vi "Terminal-Core-ModbusModule.vi"(0 "ModbusNReqRef":refnum<notifier>, 5 "ModbusNResRef":refnum<notifier>, 7 "ModbusMsgQRef":refnum<queue>, 9 "GuiModbusQRef":refnum<queue>, 11 "error in":errorcluster, 12 "ErrorQRef":refnum<queue>) -> (15 "error out":errorcluster)   [LabVIEW 2014]
panel:
  out "Exception Code":u8 format="%.0x"
  out "Holding Registers":u16[](array[numeric])
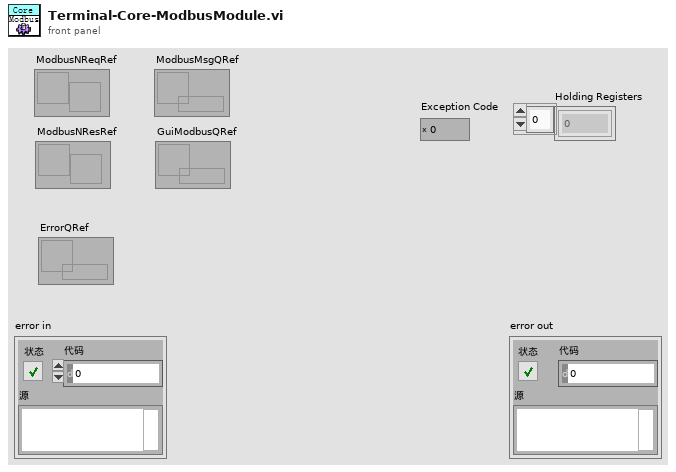
[diagram p1: front panel]
types:
  T1 = cluster{"Transaction ID":u16, "Unit ID":u8, "Starting Address":u16, "Quantity":u16}
  T2 = cluster{"Transaction ID":u16, "Unit ID":u8, "Address":u16, "Register":u16}
  T3 = cluster{"Transaction ID":u16, "Unit ID":u8, "Starting Address":u16, "Registers":u16[]}
  T4 = cluster{"Transaction ID":u16, "Unit ID":u8, "Starting Address":u16, "Quantity":u16, "Holding Registers":u16[], "Exception Code":u8}
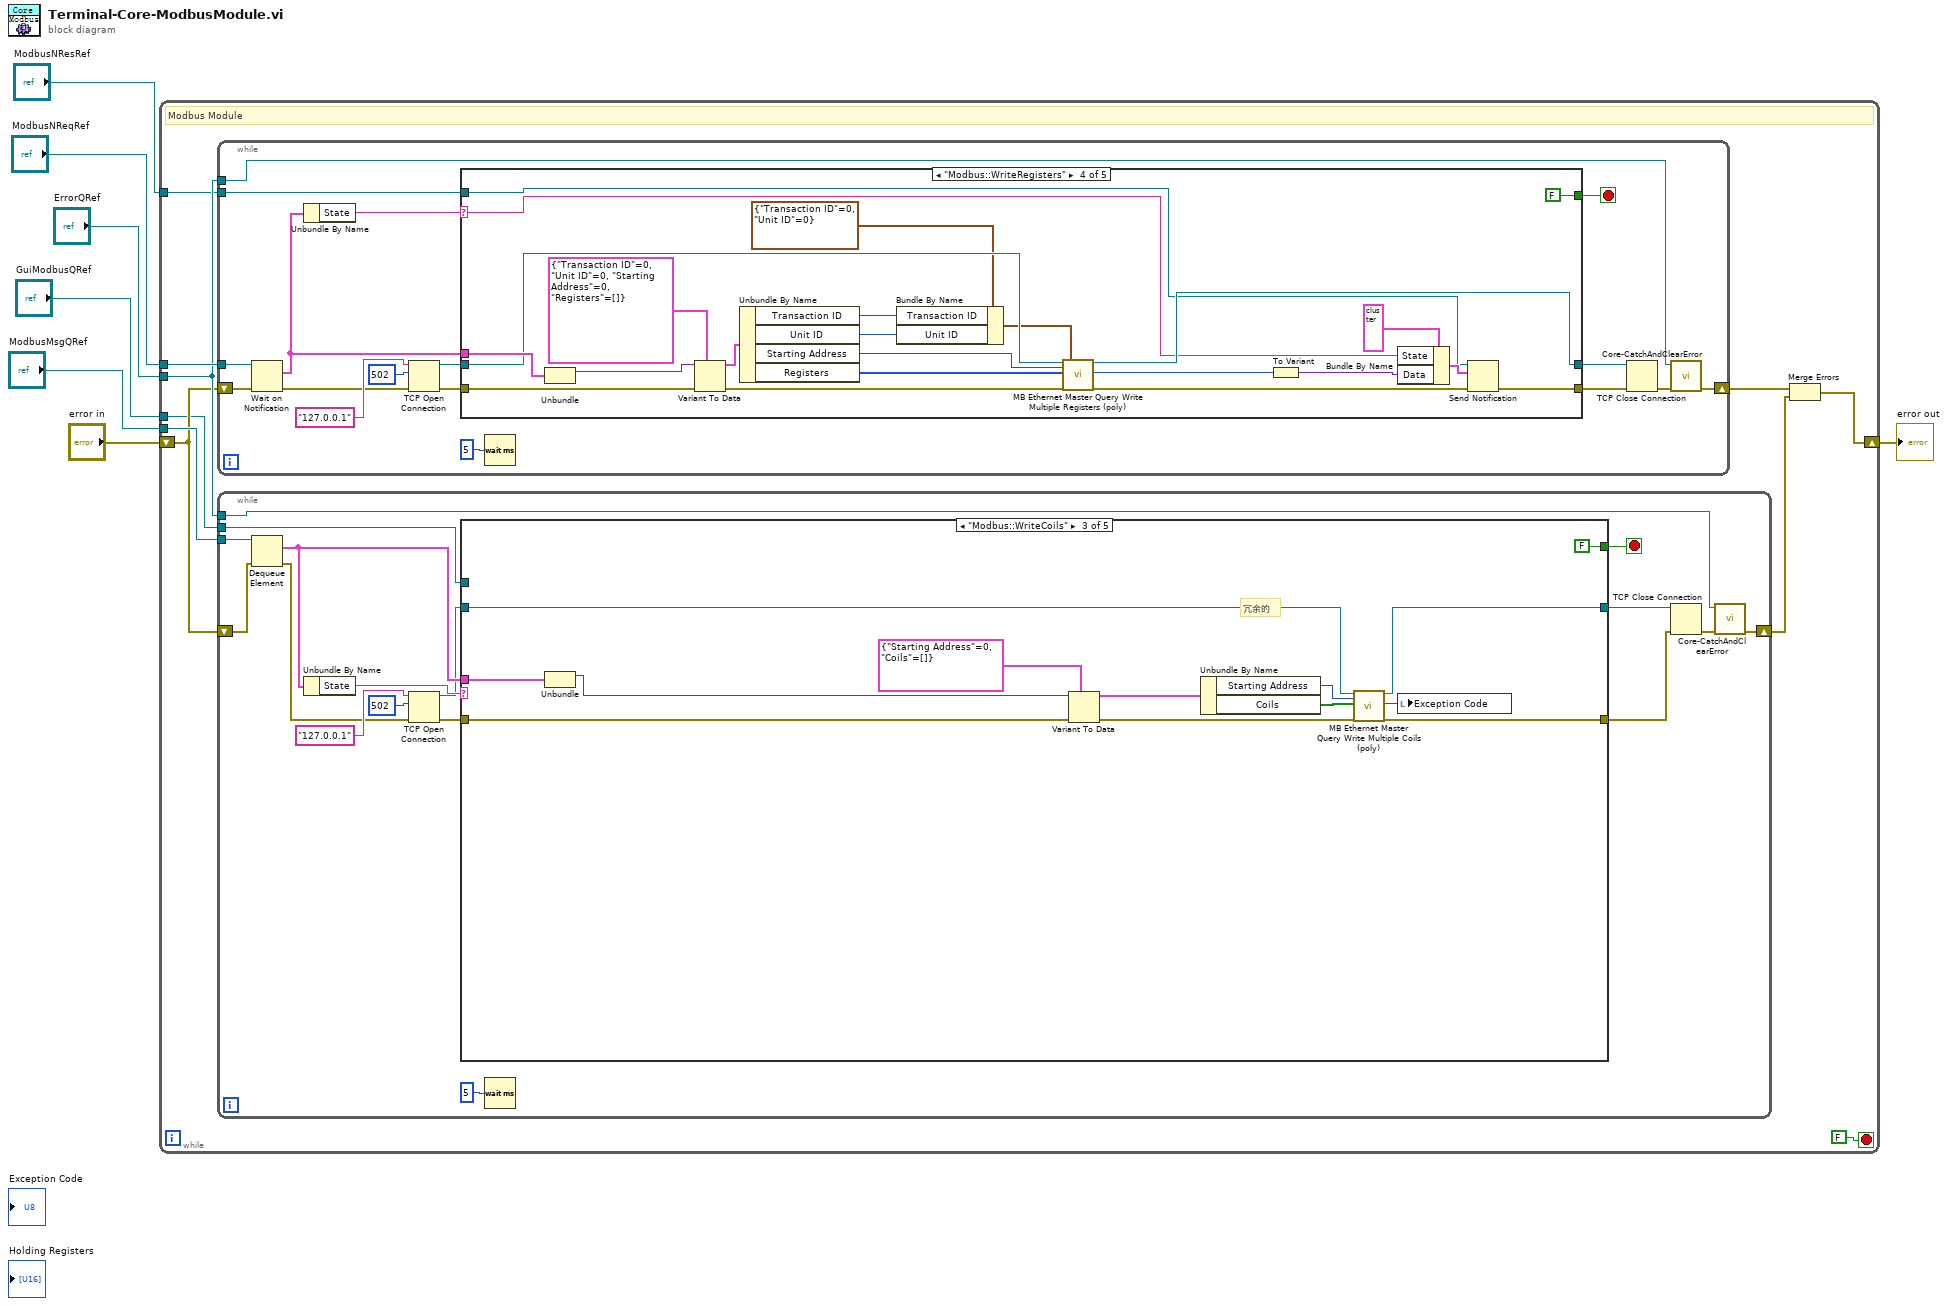
[diagram p0: block diagram]
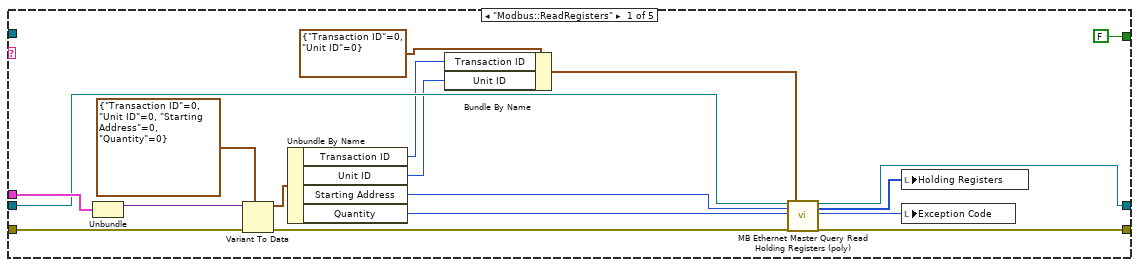
[diagram p2: hidden frame]
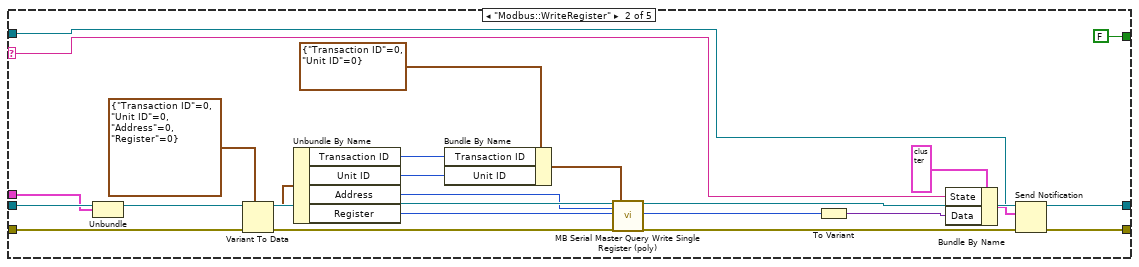
[diagram p3: hidden frame]
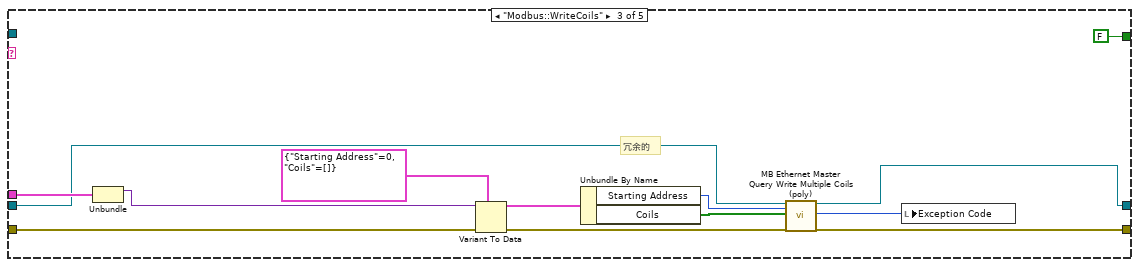
[diagram p4: hidden frame]
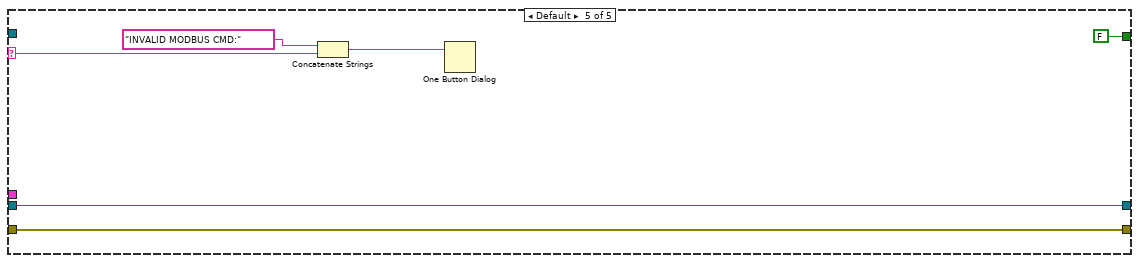
[diagram p5: hidden frame]
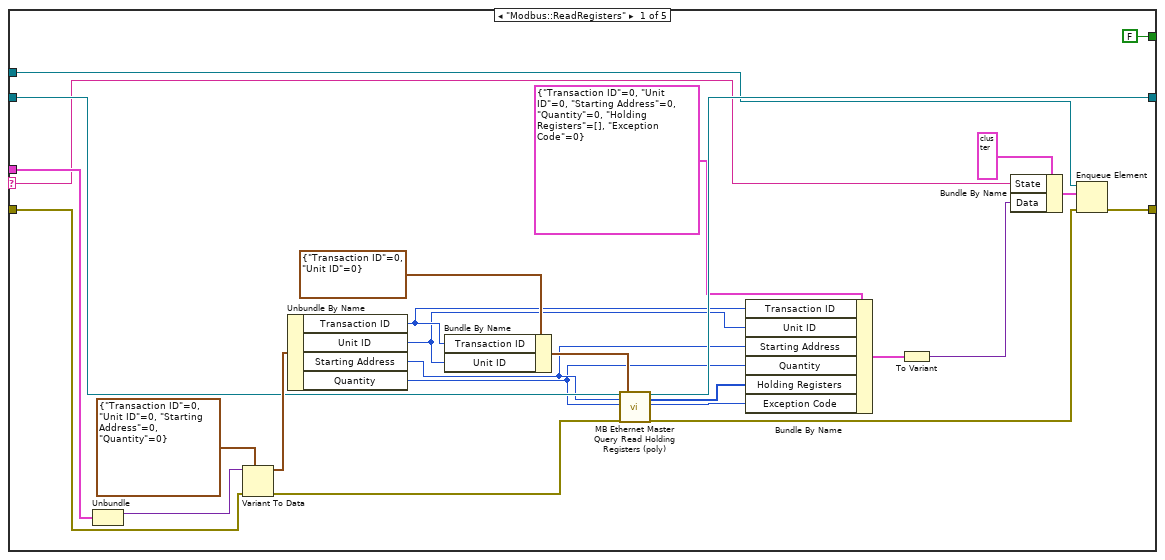
[diagram p6: hidden frame]
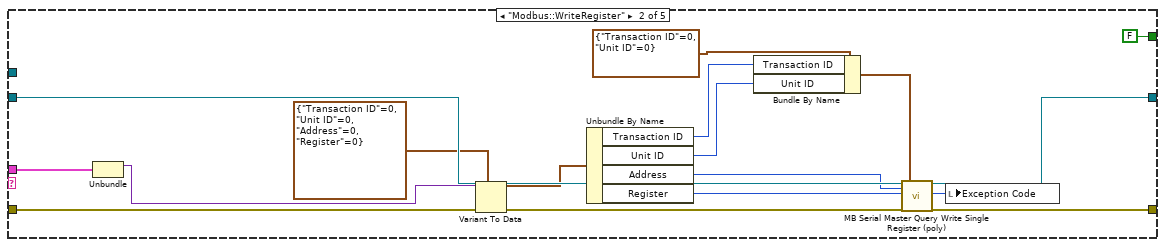
[diagram p7: hidden frame]
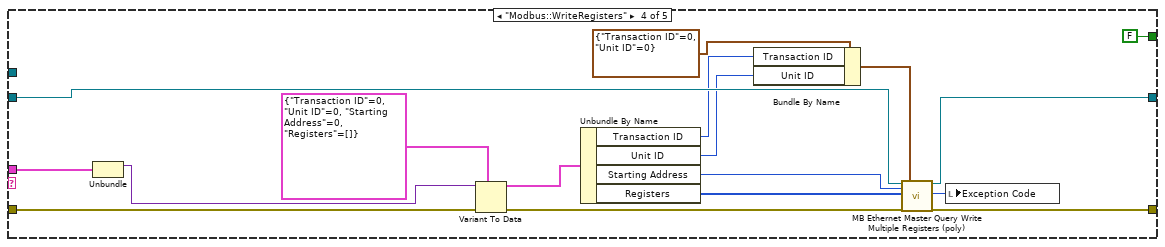
[diagram p8: hidden frame]
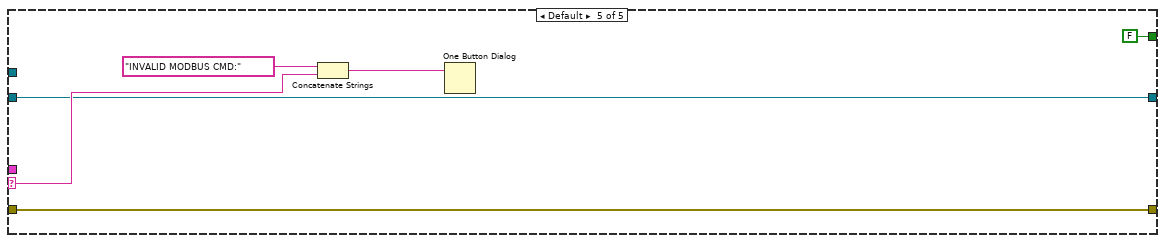
[diagram p9: hidden frame]
diagram:
  n1 = while {
    shift-right: [w8] -> w4
    shift-left: "error in" -> [w13]
    tunnel: "ErrorQRef" -> [w14]
    tunnel: "ModbusMsgQRef" -> [w17]
    tunnel: "ModbusNReqRef" -> [w15]
    tunnel: "ModbusNResRef" -> [w12]
    tunnel: "GuiModbusQRef" -> [w11]
    stop <- FALSE stop-if-true
    # "Modbus Module"
    n2 = while {
      tunnel: w14 -> [w34]
      shift-right: [w33] -> w10
      shift-left: w13 -> [w21]
      tunnel: w15 -> [w20]
      tunnel: w12 -> [w18]
      stop <- w24 stop-if-true
      n3 = Wait on Notification(notifier=w20, error in (no error)=w21) -> (notification=w19:cluster{"Data":variant, "State":string}, error out=w22:errorcluster)  [unwired: 2 in, 2 out]
      n4 = Unbundle By Name(w19) -> ("State"=w32:string)
      n5 = TCP Open Connection(address="127.0.0.1" ("地址"), remote port or service name=u16 502 ("远程端口或服务名称"), error in (no error)=w22) -> (connection ID=w28:refnum<k5>, error out=w29:errorcluster)  [unwired: 2 in]
      n6 = case shown="\"Modbus::WriteRegisters\"" w32 {
        selector: w32 -> [_ w58 _ w94 w115]
        tunnel: w19 -> [w52 w72 w87 w107 _]
        tunnel: w18 -> [_ w60 _ w91 _]
        tunnel: [FALSE FALSE FALSE FALSE FALSE] -> w24
        tunnel: w29 -> [w43 w73 w84 w106 w112]
        tunnel: w28 -> [w46 w74 w85 w104 w113]
        tunnel: [w45 w67 w81 w103 w113] -> w27
        tunnel: [w44 w54 w82 w89 w112] -> w26
        frame "Modbus::ReadRegisters" {
          n7 = Unbundle(w52) -> ("Data"=w51:variant)  [unwired: 1 out]
          n8 = Variant To Data(error in=w43, type=T1 {"Transaction ID"=0, "Unit ID"=0, "Starting Address"=0, "Quantity"=0}, Variant=w51) -> (data=w49:T1, error out=w42:errorcluster)
          n9 = Unbundle By Name(w49) -> ("Transaction ID"=w36:u16, "Unit ID"=w35:u8, "Starting Address"=w38:u16, "Quantity"=w37:u16)
          n10 = Bundle By Name(cluster=cluster{"Transaction ID":u16, "Unit ID":u8} {"Transaction ID"=0, "Unit ID"=0} ("MBAP Header"), "Transaction ID"=w36, "Unit ID"=w35) -> (w39:cluster{"Transaction ID":u16, "Unit ID":u8})
          n11 = call "MB Ethernet Master Query Read Holding Registers (poly).vi"("TCP Connection Refnum in"=w46, "Starting Address"=w38, "Quantity"=w37, "error in"=w42, "MBAP Header"=w39) -> ("TCP Connection Refnum (dup)"=w45:refnum<k5>, "Holding Registers"=w47:u16[], "Exception Code"=w48:u8, "error out"=w44:errorcluster)  [unwired: 11 in]
          n12 = local write "Holding Registers"(w47) -> ()
          n13 = local write "Exception Code"(w48) -> ()
        }
        frame "Modbus::WriteRegister" {
          n14 = Unbundle(w72) -> ("Data"=w71:variant)  [unwired: 1 out]
          n15 = Variant To Data(error in=w73, type=T2 {"Transaction ID"=0, "Unit ID"=0, "Address"=0, "Register"=0}, Variant=w71) -> (data=w69:T2, error out=w68:errorcluster)
          n16 = Unbundle By Name(w69) -> ("Transaction ID"=w64:u16, "Unit ID"=w63:u8, "Address"=w62:u16, "Register"=w61:u16)
          n17 = Bundle By Name(cluster=cluster{"Transaction ID":u16, "Unit ID":u8} {"Transaction ID"=0, "Unit ID"=0} ("MBAP Header"), "Transaction ID"=w64, "Unit ID"=w63) -> (w65:cluster{"Transaction ID":u16, "Unit ID":u8})
          n18 = call "MB Serial Master Query Write Single Register (poly).vi"("VISA resource name"=w74, "Address"=w62, "Holding Register"=w61, "error in"=w68, "Serial Parameters"=w65) -> ("VISA resource name out"=w67:refnum<visa-resource-name>, "Exception Code"=w57:u8, "error out"=w55:errorcluster)  [unwired: 12 in]
          n19 = To Variant(anything=w57) -> (Variant=w56:variant)
          n20 = Bundle By Name(cluster=cluster{"Data":variant, "State":string} {"Data"=variant, "State"=""} ("通知"), "State"=w58, "Data"=w56) -> (w53:cluster{"Data":variant, "State":string})
          n21 = Send Notification(notification=w53, notifier=w60, error in (no error)=w55) -> (error out=w54:errorcluster)  [unwired: 1 out]
        }
        frame "Modbus::WriteCoils" {
          # "冗余的"
          n22 = Unbundle(w87) -> ("Data"=w86:variant)  [unwired: 1 out]
          n23 = Variant To Data(error in=w84, type=cluster{"Starting Address":u16, "Coils":bool[]} {"Starting Address"=0, "Coils"=[]}, Variant=w86) -> (data=w78:cluster{"Starting Address":u16, "Coils":bool[]}, error out=w83:errorcluster)
          n24 = Unbundle By Name(w78) -> ("Starting Address"=w77:u16, "Coils"=w76:bool[])
          n25 = call "MB Ethernet Master Query Write Multiple Coils (poly).vi"("TCP Connection Refnum in"=w85, "Starting Address"=w77, "Coils"=w76, "error in"=w83) -> ("TCP Connection Refnum (dup)"=w81:refnum<k5>, "Exception Code"=w80:u8, "error out"=w82:errorcluster)  [unwired: 13 in]
          n26 = local write "Exception Code"(w80) -> ()
        }
        frame "Modbus::WriteRegisters" {
          n27 = Unbundle(w107) -> ("Data"=w110:variant)  [unwired: 1 out]
          n28 = Variant To Data(error in=w106, type=T3 {"Transaction ID"=0, "Unit ID"=0, "Starting Address"=0, "Registers"=[]}, Variant=w110) -> (data=w108:T3, error out=w105:errorcluster)
          n29 = Unbundle By Name(w108) -> ("Transaction ID"=w99:u16, "Unit ID"=w98:u8, "Starting Address"=w101:u16, "Registers"=w102:u16[])
          n30 = Bundle By Name(cluster=cluster{"Transaction ID":u16, "Unit ID":u8} {"Transaction ID"=0, "Unit ID"=0} ("MBAP Header"), "Transaction ID"=w99, "Unit ID"=w98) -> (w97:cluster{"Transaction ID":u16, "Unit ID":u8})
          n31 = call "MB Ethernet Master Query Write Multiple Registers (poly).vi"("TCP Connection Refnum in"=w104, "Starting Address"=w101, "Registers"=w102, "error in"=w105, "MBAP Header"=w97) -> ("TCP Connection Refnum (dup)"=w103:refnum<k5>, "Exception Code"=w96:u8, "error out"=w90:errorcluster)  [unwired: 12 in]
          n32 = To Variant(anything=w96) -> (Variant=w95:variant)
          n33 = Bundle By Name(cluster=cluster{"Data":variant, "State":string} {"Data"=variant, "State"=""} ("通知"), "State"=w94, "Data"=w95) -> (w92:cluster{"Data":variant, "State":string})
          n34 = Send Notification(notification=w92, notifier=w91, error in (no error)=w90) -> (error out=w89:errorcluster)  [unwired: 1 out]
        }
        frame Default {
          n35 = Concatenate Strings("INVALID MODBUS CMD:", w115) -> (w116:string)
          n36 = One Button Dialog(message=w116) -> ()  [unwired: 1 in, 1 out]
        }
      }
      n37 = Wait (ms)(milliseconds to wait=u32 5 ("等待时间（毫秒）")) -> ()  [unwired: 1 out]
      n38 = TCP Close Connection(connection ID=w27, error in (no error)=w26) -> (error out=w25:errorcluster)  [unwired: 1 in, 1 out]
      n39 = call "Core-CatchAndClearError.vi"("error in (no error)"=w25, "ErrorQ"=w34) -> ("error out"=w33:errorcluster)  [unwired: 7 in]
    }
    n40 = while {
      tunnel: w17 -> [w134]
      tunnel: w14 -> [w132]
      shift-right: [w131] -> w9
      shift-left: w13 -> [w133]
      tunnel: w11 -> [w118]
      stop <- w120 stop-if-true
      n41 = Dequeue Element(queue=w134, error in (no error)=w133) -> (element=w129:cluster{"Data":variant, "State":string}, error out=w126:errorcluster)  [unwired: 1 in, 2 out]
      n42 = Unbundle By Name(w129) -> ("State"=w130:string)
      n43 = TCP Open Connection(address="127.0.0.1" ("地址"), remote port or service name=u16 502 ("远程端口或服务名称"), error in (no error)=w126) -> (connection ID=w124:refnum<k5>, error out=w125:errorcluster)  [unwired: 2 in]
      n44 = case shown="\"Modbus::WriteCoils\"" w130 {
        selector: w130 -> [w145 _ _ _ w211]
        tunnel: w129 -> [w160 w174 w189 w203 _]
        tunnel: [FALSE FALSE FALSE FALSE FALSE] -> w120
        tunnel: w125 -> [w154 w175 w186 w202 w208]
        tunnel: w124 -> [w156 w176 w187 w199 w209]
        tunnel: [w155 w167 w183 w198 w209] -> w123
        tunnel: [w140 w169 w184 w200 w208] -> w122
        tunnel: w118 -> [w149 _ _ _ _]
        frame "Modbus::ReadRegisters" {
          n45 = Unbundle(w160) -> ("Data"=w159:variant)  [unwired: 1 out]
          n46 = Variant To Data(error in=w154, type=T1 {"Transaction ID"=0, "Unit ID"=0, "Starting Address"=0, "Quantity"=0}, Variant=w159) -> (data=w157:T1, error out=w153:errorcluster)
          n47 = Unbundle By Name(w157) -> ("Transaction ID"=w138:u16, "Unit ID"=w137:u8, "Starting Address"=w136:u16, "Quantity"=w135:u16)
          n48 = Bundle By Name(cluster=cluster{"Transaction ID":u16, "Unit ID":u8} {"Transaction ID"=0, "Unit ID"=0} ("MBAP Header"), "Transaction ID"=w138, "Unit ID"=w137) -> (w150:cluster{"Transaction ID":u16, "Unit ID":u8})
          n49 = call "MB Ethernet Master Query Read Holding Registers (poly).vi"("TCP Connection Refnum in"=w156, "Starting Address"=w136, "Quantity"=w135, "error in"=w153, "MBAP Header"=w150) -> ("TCP Connection Refnum (dup)"=w155:refnum<k5>, "Holding Registers"=w139:u16[], "Exception Code"=w143:u8, "error out"=w141:errorcluster)  [unwired: 11 in]
          n50 = Bundle By Name(cluster=T4 {"Transaction ID"=0, "Unit ID"=0, "Starting Address"=0, "Quantity"=0, "Holding Registers"=[], "Exception Code"=0} ("元素"), "Transaction ID"=w138, "Unit ID"=w137, "Starting Address"=w136, "Quantity"=w135, "Holding Registers"=w139, "Exception Code"=w143) -> (w147:T4)
          n51 = To Variant(anything=w147) -> (Variant=w146:variant)
          n52 = Bundle By Name(cluster=cluster{"Data":variant, "State":string} {"Data"=variant, "State"=""} ("元素"), "State"=w145, "Data"=w146) -> (w142:cluster{"Data":variant, "State":string})
          n53 = Enqueue Element(queue=w149, element=w142, error in (no error)=w141) -> (error out=w140:errorcluster)  [unwired: 1 in, 2 out]
        }
        frame "Modbus::WriteRegister" {
          n54 = Unbundle(w174) -> ("Data"=w173:variant)  [unwired: 1 out]
          n55 = Variant To Data(error in=w175, type=T2 {"Transaction ID"=0, "Unit ID"=0, "Address"=0, "Register"=0}, Variant=w173) -> (data=w171:T2, error out=w170:errorcluster)
          n56 = Unbundle By Name(w171) -> ("Transaction ID"=w164:u16, "Unit ID"=w163:u8, "Address"=w162:u16, "Register"=w161:u16)
          n57 = Bundle By Name(cluster=cluster{"Transaction ID":u16, "Unit ID":u8} {"Transaction ID"=0, "Unit ID"=0} ("MBAP Header"), "Transaction ID"=w164, "Unit ID"=w163) -> (w165:cluster{"Transaction ID":u16, "Unit ID":u8})
          n58 = call "MB Serial Master Query Write Single Register (poly).vi"("VISA resource name"=w176, "Address"=w162, "Holding Register"=w161, "error in"=w170, "Serial Parameters"=w165) -> ("VISA resource name out"=w167:refnum<visa-resource-name>, "Exception Code"=w168:u8, "error out"=w169:errorcluster)  [unwired: 12 in]
          n59 = local write "Exception Code"(w168) -> ()
        }
        frame "Modbus::WriteCoils" {
          # "冗余的"
          n60 = Unbundle(w189) -> ("Data"=w188:variant)  [unwired: 1 out]
          n61 = Variant To Data(error in=w186, type=cluster{"Starting Address":u16, "Coils":bool[]} {"Starting Address"=0, "Coils"=[]}, Variant=w188) -> (data=w180:cluster{"Starting Address":u16, "Coils":bool[]}, error out=w185:errorcluster)
          n62 = Unbundle By Name(w180) -> ("Starting Address"=w179:u16, "Coils"=w178:bool[])
          n63 = call "MB Ethernet Master Query Write Multiple Coils (poly).vi"("TCP Connection Refnum in"=w187, "Starting Address"=w179, "Coils"=w178, "error in"=w185) -> ("TCP Connection Refnum (dup)"=w183:refnum<k5>, "Exception Code"=w182:u8, "error out"=w184:errorcluster)  [unwired: 13 in]
          n64 = local write "Exception Code"(w182) -> ()
        }
        frame "Modbus::WriteRegisters" {
          n65 = Unbundle(w203) -> ("Data"=w206:variant)  [unwired: 1 out]
          n66 = Variant To Data(error in=w202, type=T3 {"Transaction ID"=0, "Unit ID"=0, "Starting Address"=0, "Registers"=[]}, Variant=w206) -> (data=w204:T3, error out=w201:errorcluster)
          n67 = Unbundle By Name(w204) -> ("Transaction ID"=w193:u16, "Unit ID"=w192:u8, "Starting Address"=w195:u16, "Registers"=w196:u16[])
          n68 = Bundle By Name(cluster=cluster{"Transaction ID":u16, "Unit ID":u8} {"Transaction ID"=0, "Unit ID"=0} ("MBAP Header"), "Transaction ID"=w193, "Unit ID"=w192) -> (w191:cluster{"Transaction ID":u16, "Unit ID":u8})
          n69 = call "MB Ethernet Master Query Write Multiple Registers (poly).vi"("TCP Connection Refnum in"=w199, "Starting Address"=w195, "Registers"=w196, "error in"=w201, "MBAP Header"=w191) -> ("TCP Connection Refnum (dup)"=w198:refnum<k5>, "Exception Code"=w197:u8, "error out"=w200:errorcluster)  [unwired: 12 in]
          n70 = local write "Exception Code"(w197) -> ()
        }
        frame Default {
          n71 = Concatenate Strings("INVALID MODBUS CMD:", w211) -> (w212:string)
          n72 = One Button Dialog(message=w212) -> ()  [unwired: 1 in, 1 out]
        }
      }
      n73 = Wait (ms)(milliseconds to wait=u32 5 ("等待时间（毫秒）")) -> ()  [unwired: 1 out]
      n74 = TCP Close Connection(connection ID=w123, error in (no error)=w122) -> (error out=w121:errorcluster)  [unwired: 1 in, 1 out]
      n75 = call "Core-CatchAndClearError.vi"("error in (no error)"=w121, "ErrorQ"=w132) -> ("error out"=w131:errorcluster)  [unwired: 7 in]
    }
    n76 = Merge Errors(w10, w9) -> (w8:errorcluster)
  }
  "error out" <- w4
